vi "Prepare stdin.vi"(8 "error in (no error)":errorcluster, 10 "FileCopy Job Config":T1, 11 "Job.SingleFileCopy in":refnum<class "Job.SingleFileCopy.lvclass">) -> (0 "error out":errorcluster, 2 "Stdin":string, 3 "Job.SingleFileCopy out":refnum<class "Job.SingleFileCopy.lvclass">)   [LabVIEW 2013, in "Job.SingleFileCopy.lvclass"]
uses:
  Job.SingleFileCopy.lvclass
  FileCopy Job Configuration -- cluster.ctl
  <vilib>/addons/_JKI.lib/Serialization/JSON/JKI JSON Serialization.lvlib
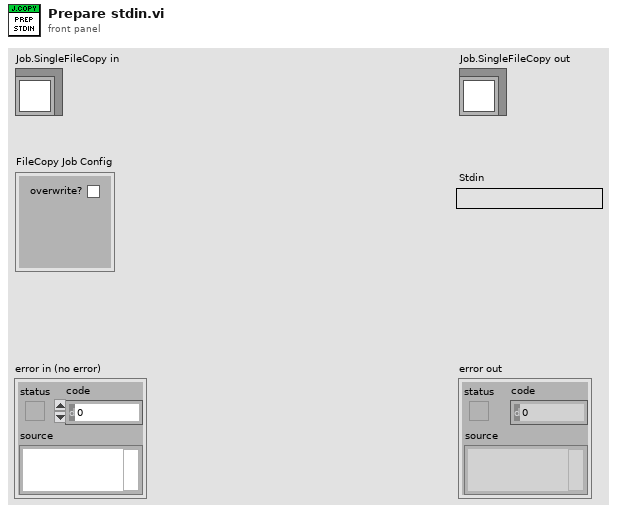
[diagram p1: front panel]
types:
  T1 = typedef "Job.SingleFileCopy.lvclass/FileCopy Job Configuration -- cluster.ctl" = cluster{"overwrite?":bool}
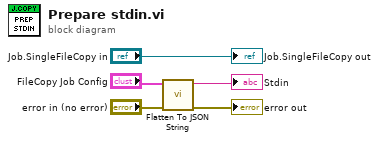
[diagram p0: block diagram]
diagram:
  n1 = call <vilib>:"Flatten To JSON String.vi"("error in (no error)"="error in (no error)", "Variant"="FileCopy Job Config") -> ("error out"=→"error out":errorcluster, "JSON String"=→"Stdin":string)  [unwired: 8 in]
  "Job.SingleFileCopy out" <- "Job.SingleFileCopy in"
